vi "Plot menu selection.vi"(8 "error in (no error)":errorcluster, 10 "ItemTag":string, 11 "BluePlotHandle in":refnum<class "BluePlotHandle.lvclass">) -> (0 "error out":errorcluster, 3 "BluePlotHandle out":refnum<class "BluePlotHandle.lvclass">)   [LabVIEW 2021, in "BluePlot.lvlib" / "BluePlotHandle.lvclass"]
uses:
  BluePlotHandle.lvclass
  BluePlotHandle.lvclass/BluePlotHandle.ctl
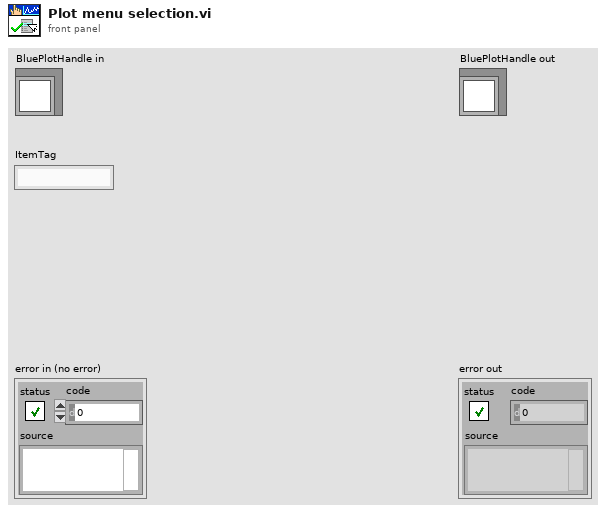
[diagram p1: front panel]
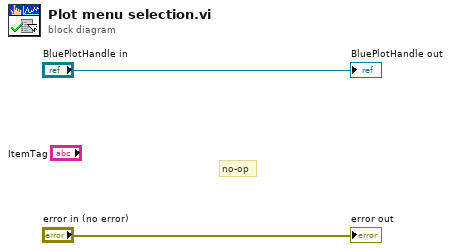
[diagram p0: block diagram]
diagram:
  # "no-op"
  "error out" <- "error in (no error)"
  "BluePlotHandle out" <- "BluePlotHandle in"
